vi "Read I64 4.vi"(8 "error in (no error)":errorcluster, 11 "CIFTemplateNode in":refnum<class "CIFCorePlugin.lvclass">) -> (0 "error out":errorcluster, 2 "i64":i64, 3 "CIFTemplateNode out":refnum<class "CIFCorePlugin.lvclass">)   [LabVIEW 2021, in "CIFCorePlugin.lvclass"]
uses:
  CIFCorePlugin.lvclass
  CIFCorePlugin.lvclass/CIFCorePlugin.ctl
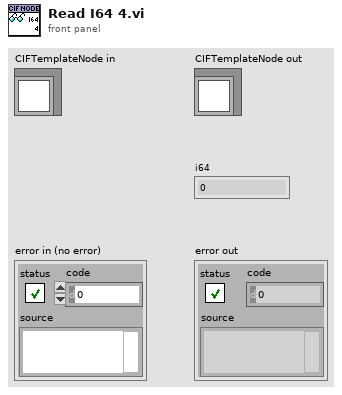
[diagram p1: front panel]
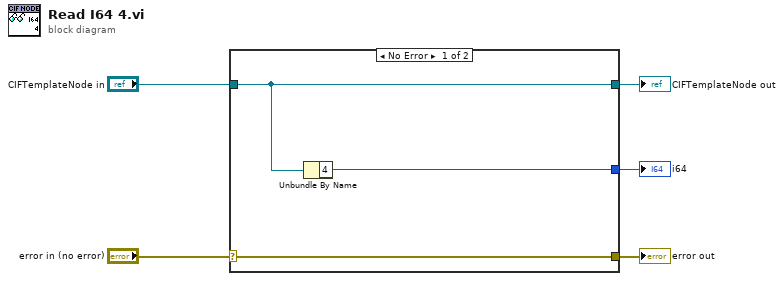
[diagram p0: block diagram]
diagram:
  n1 = case shown="No Error" "error in (no error)" {
    selector: "error in (no error)" -> [w8 w9]
    tunnel: [w8 w9] -> w4
    tunnel: [w7 w10] -> w2
    tunnel: "CIFTemplateNode in" -> [w7 w10]
    tunnel: [w6 _] -> w1
    frame No Error {
      n2 = Unbundle By Name(w7) -> ("4"=w6:i64)
    }
    frame Error {
    }
  }
  "error out" <- w4
  "CIFTemplateNode out" <- w2
  "i64" <- w1
